vi "MGI Handle Row Select.vi"(8 "error in (no error)":errorcluster, 9 "Old Selected[]":i32[](array[numeric]), 10 "Selected[]":i32[](array[numeric]), 11 "MGI Error Handler in":refnum<class "MGI Error Reporter Dialog.lvclass">) -> (0 "error out":errorcluster, 3 "MGI Error Handler out":refnum<class "MGI Error Reporter Dialog.lvclass">)   [LabVIEW 2020, in "MGI Error Reporter Dialog.lvclass"]
doc: "Handle actions associated with selecting a new row in the Error History listbox. The Call Chain Ring and Details String controls are updated with information for the selected error, or disabled if there is no error selected. The MGI Error Handler only supports one error selected at a time, but this VI uses an array so that a child class may override this behavior.\n\nAuthored by Shawn Walpole\nsupport@mooregoodideas.com\nwww.mooregoodideas.com\n\nCopyright (c) 2010, Moore Good Ideas, Inc.\n\nAll rights reserved.\n\nRedistribution and use in source and binary forms, with or without modification, are permitted provided that the following conditions are met:\n\n * Redistributions of source code must retain the above copyright notice, this list of conditions and the following disclaimer.\n * Redistributions in binary form must reproduce the above copyright notice, this list of conditions and the following disclaimer in the documentation and/or other materials provided with the distribution.\n * Neither the name of Moore Good Ideas, Inc. nor the names of its contributors may be used to endorse or promote products derived from this software without specific prior written permission.\n\nTHIS SOFTWARE IS PROVIDED BY THE COPYRIGHT HOLDERS AND CONTRIBUTORS \"AS IS\" AND ANY EXPRESS OR IMPLIED WARRANTIES, INCLUDING, BUT NOT LIMITED TO, THE IMPLIED WARRANTIES OF MERCHANTABILITY AND FITNESS FOR A PARTICULAR PURPOSE ARE DISCLAIMED. IN NO EVENT SHALL THE COPYRIGHT OWNER OR CONTRIBUTORS BE LIABLE FOR ANY DIRECT, INDIRECT, INCIDENTAL, SPECIAL, EXEMPLARY, OR CONSEQUENTIAL DAMAGES (INCLUDING, BUT NOT LIMITED TO, PROCUREMENT OF SUBSTITUTE GOODS OR SERVICES; LOSS OF USE, DATA, OR PROFITS; OR BUSINESS INTERRUPTION) HOWEVER CAUSED AND ON ANY THEORY OF LIABILITY, WHETHER IN CONTRACT, STRICT LIABILITY, OR TORT (INCLUDING NEGLIGENCE OR OTHERWISE) ARISING IN ANY WAY OUT OF THE USE OF THIS SOFTWARE, EVEN IF ADVISED OF THE POSSIBILITY OF SUCH DAMAGE."
uses:
  <userlib>/_MGI/Error Reporter/MGI Error Reporter Dialog/MGI Error Reporter Dialog.lvclass
  <userlib>/_MGI/Error Reporter/MGI Error Reporter Dialog/MGI Error Reporter Dialog.lvclass/MGI Error Reporter Dialog.ctl
  <userlib>/_MGI/Application Control/MGI Gray if/MGI Gray if True.vi
  <userlib>/_MGI/Application Control/MGI Set Scrollbar/MGI Set String Scrollbar.vi
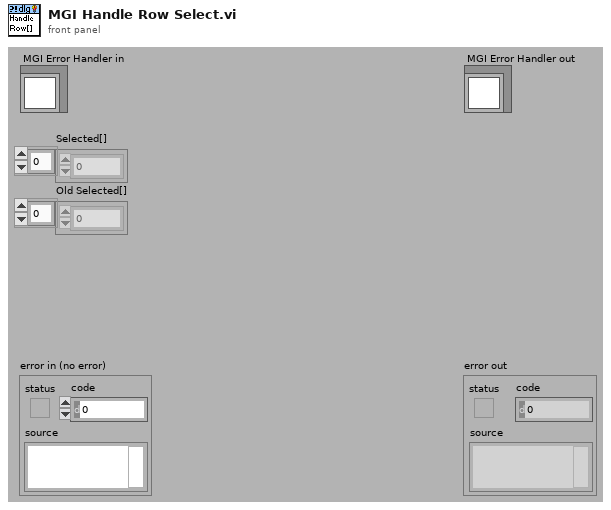
[diagram p1: front panel]
types:
  T1 = enum8{"Enabled", "Disabled", "Disabled and Grayed Out"}
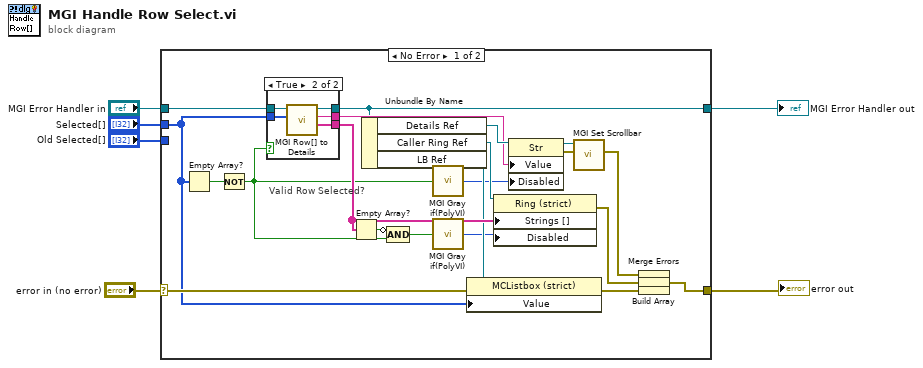
[diagram p0: block diagram]
diagram:
  n1 = case shown="No Error" "error in (no error)" {
    selector: "error in (no error)" -> [w16 w36]
    tunnel: [w23 w36] -> w5
    tunnel: [w24 w35] -> w3
    tunnel: "MGI Error Handler in" -> [w25 w35]
    tunnel: "Selected[]" -> [w15 _]
    tunnel: "Old Selected[]" -> [_ _]
    frame No Error {
      # "Valid Row Selected?"
      n2 = Empty Array?(array=w15) -> (empty?=w18:bool)
      n3 = Not(x=w18) -> (.not. x?=w10:bool)
      n4 = case shown="True" w10 {
        tunnel: [_ w32] -> w26
        tunnel: [_ w31] -> w22
        tunnel: [w29 w33] -> w24
        tunnel: w25 -> [w29 w34]
        tunnel: w15 -> [_ w30]
        frame False {
        }
        frame True {
          n5 = call-dynamic "MGI Row[] to Details.vi"("Selected Row[]"=w30, "MGI Error Reporter Dialog In"=w34) -> ("Call Chain[occurred..TopLevel]"=w31:string[], "Error Details"=w32:string, "MGI Error Reporter Dialog Out"=w33:refnum<class "MGI Error Reporter Dialog.lvclass">)  [unwired: 7 out]
        }
      }
      n6 = Empty Array?(array=w22) -> (empty?=w21:bool)
      n7 = Unbundle By Name(w24) -> ("Details Ref"=w28:refnum<vi>, "Caller Ring Ref"=w27:refnum<vi>, "LB Ref"=w17:refnum<vi>)
      n8 = Compound Arithmetic op=AND(invert w21, w10) -> (w8:bool)
      n9 = call-poly <userlib>:"MGI Gray if(PolyVI).vi"("True?"=w10) -> ("Disabled"=w9:T1)
      n10 = call-poly <userlib>:"MGI Gray if(PolyVI).vi"("True?"=w8) -> ("Disabled"=w7:T1)
      n11 = property class="MCListbox (strict)"(reference=w17, error in=w16, "Value"=w15) -> (error out=w12:errorcluster)  [unwired: 1 out]
      n12 = property class="Ring (strict)"(reference=w27, "Strings []"=w22, "Disabled"=w7) -> (error out=w13:errorcluster)  [unwired: 1 in, 1 out]
      n13 = property class="Str"(reference=w28, "Value"=w26, "Disabled"=w9) -> (reference out=w20:refnum<vi>, error out=w19:errorcluster)  [unwired: 1 in]
      n14 = call-poly <userlib>:"MGI Set Scrollbar.vi"("Error In"=w19, "String Reference"=w20) -> ("Error Out"=w14:errorcluster)  [unwired: 9 out]
      n15 = Build Array(w14, w13, w12) -> (w11:errorcluster[])
      n16 = Merge Errors(w11) -> (w23:errorcluster)
    }
    frame Error {
    }
  }
  "error out" <- w5
  "MGI Error Handler out" <- w3
